vi "Main_001.vi"() -> ()   [LabVIEW 2025]
uses:
  Utility/Universal Utility/TypeDefs_Utility/Cluster_Row-Column.ctl
  9e3f57c0-2ef8-4495-8287-c6a42a5fb955.vi
  Utility/Universal Utility/TypeDefs_Utility/ENUM_4 Directions U-D-L-R.ctl
  Utility/Universal Utility/TypeDefs_Utility/ENUM_8 Directions U-D-L-R.ctl
panel:
  out "Array":i32[](array[numeric])
  out "MATCH":bool
  in  "Select Data":enum32{"Example", "Puzzle"}(tab)
  in  "EX Natural Numbers below that are\nmultiples of 3 or 5":u64=1000
  in  "EX Target":u64=233168
  in  "Natural Numbers below that are\nmultiples of 3 or 5":u64=10
  in  "Target":u64=23
  out "Answer":u64
  # "https://projecteuler.net/problem=1"
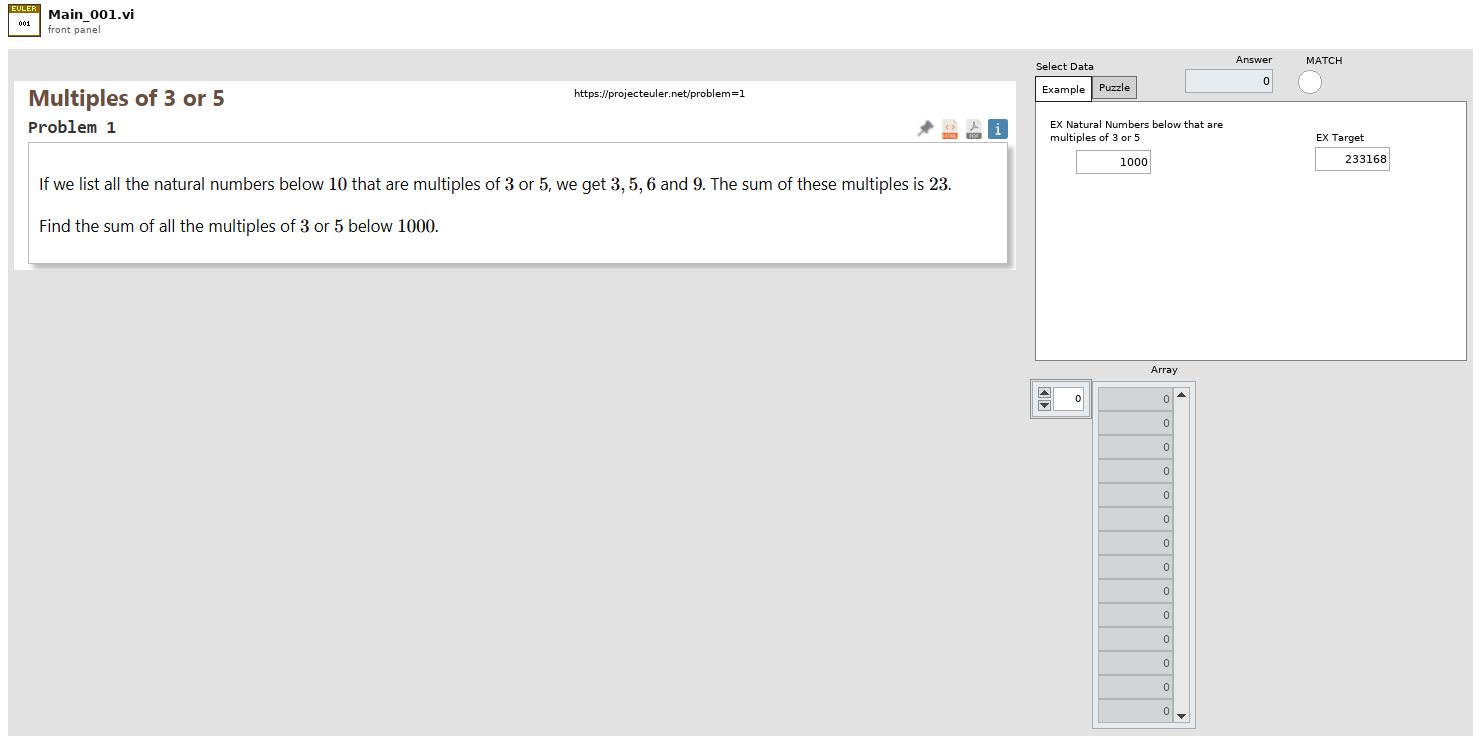
[diagram p1: front panel]
types:
  T1 = typedef "ENUM_8 Directions U-D-L-R.ctl" = enum16{"Up;-1,0", "Up-Right;-1,1", "Right;0,1", "Down-Right;1,1", "Down;1,0", "Down-Left;1,-1", "Left;0,-1", "Up-Left;-1,-1"}
  T2 = typedef "ENUM_4 Directions U-D-L-R.ctl" = enum16{"Up;-1,0", "Right;0,1", "Down;1,0", "Left;0,-1"}
  T3 = typedef "Cluster_Row-Column.ctl" = cluster{"R":i32, "C":i32}
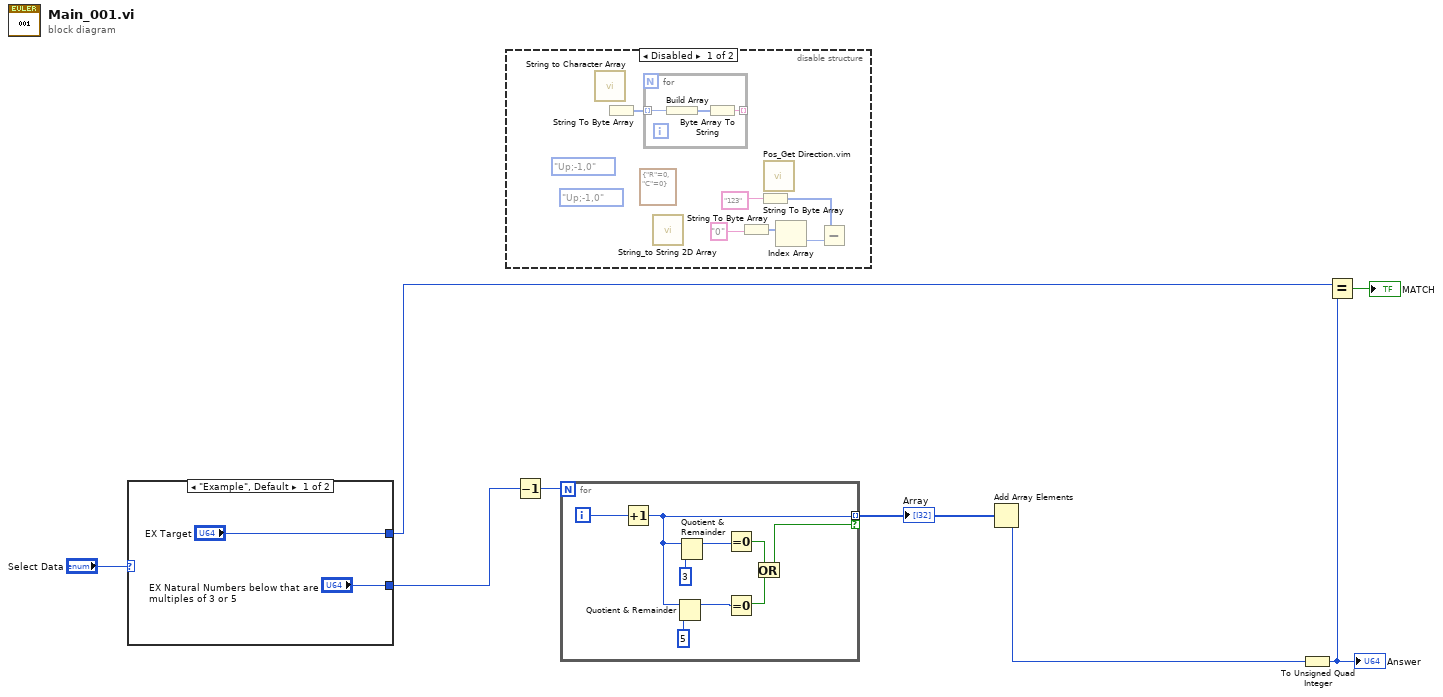
[diagram p0: block diagram]
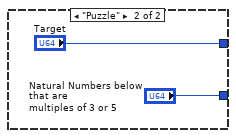
[diagram p2: hidden frame]
diagram:
  n1 = case shown="\"Example\", Default" "Select Data" {
    tunnel: ["EX Target" "Target"] -> w6
    tunnel: ["EX Natural Numbers below that are\nmultiples of 3 or 5" "Natural Numbers below that are\nmultiples of 3 or 5"] -> w4
    frame "Example", Default {
    }
    frame "Puzzle" {
    }
  }
  n2 = disable-structure shown="Disabled" {
    frame Disabled {
      (unwired) ENUM_8_Directions_U-D-L-R."Up;-1,0" ("Direction 8")
      (unwired) ENUM_4_Directions_U-D-L-R."Up;-1,0" ("Direction")
      (unwired) T3 {"R"=0, "C"=0} ("Position")
      n3 = call "String to Character Array.vi"() -> ()  [unwired: 1 in, 1 out]
      n4 = String To Byte Array() -> (unsigned byte array=w13:u8[])  [unwired: 1 in]
      n5 = for {
        tunnel: w13 -> [w21] mode=indexing
        tunnel: [w19] -> _ mode=indexing
        n6 = Build Array(w21) -> (w20:u8[])
        n7 = Byte Array To String(unsigned byte array=w20) -> (string=w19:string)
      }
      n8 = call "String_to String 2D Array.vi"() -> ()  [unwired: 11 in, 1 out]
      n9 = String To Byte Array(string="0") -> (unsigned byte array=w16:u8[])
      n10 = String To Byte Array(string="123") -> (unsigned byte array=w14:u8[])
      n11 = call "Pos_Get Direction.vim"() -> ()  [unwired: 11 in, 1 out]
      n12 = Index Array(array=w16) -> (element=w15:u8)  [unwired: 1 in]
      n13 = Subtract(x=w14, y=w15) -> ()  [unwired: 1 out]
    }
    frame Enabled {
    }
  }
  n14 = Decrement(x=w4) -> (x-1=w3:u64)
  n15 = for {
    N: w3 -> [_]
    tunnel: [w29] -> w2 mode=indexing if=w24
    i -> [w30]
    n16 = Increment(x=w30) -> (x+1=w29:i32)
    n17 = Quotient & Remainder(x=w29, y=5) -> (x-y*floor(x/y)=w27:i32)  [unwired: 1 out]
    n18 = Quotient & Remainder(x=w29, y=3) -> (x-y*floor(x/y)=w28:i32)  [unwired: 1 out]
    n19 = Equal To 0?(x=w28) -> (x = 0?=w26:bool)
    n20 = Equal To 0?(x=w27) -> (x = 0?=w25:bool)
    n21 = Or(x=w26, y=w25) -> (x .or. y?=w24:bool)
  }
  "Array" <- w2
  n22 = Add Array Elements(numeric array=w2) -> (sum=w1:i32)
  n23 = To Unsigned Quad Integer(1:w1) -> (0:w5:u64)
  "Answer" <- w5
  n24 = Equal?(x=w6, y=w5) -> (x = y?=→"MATCH":bool)
